vi "Com_Lookup.vi"(8 "Fehler (Eingang, kein Fehler)":errorcluster) -> (0 "Fehler (Ausgang)":errorcluster, 3 "find list":string[](array[string]))   [LabVIEW 2020, in "Linearisierung v2.lvlib" / "Gasteiler.lvlib" / "HovaCAL_Interface.lvlib" / "Helper.lvlib"]
uses:
  Helper.lvlib
  <vilib>/Instr/_visa.llb/VISA Find Search Mode.ctl
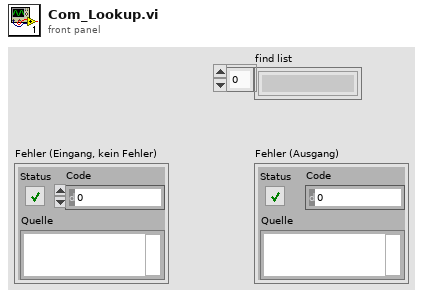
[diagram p1: front panel]
types:
  T1 = typedef "VISA Find Search Mode.ctl" = u32
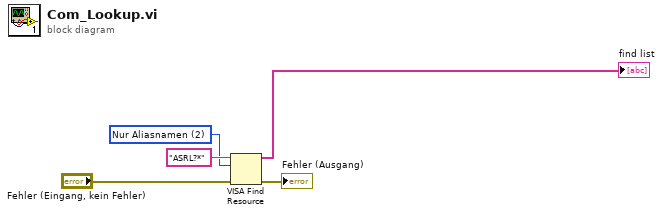
[diagram p0: block diagram]
diagram:
  w3 = T1 2 items=["Nur anerkannte Namen"=0, "Nur Aliasnamen"=2, "Übereinstimmende Aliasnamen einschließen"=3, "Alle Aliasnamen einschließen"=4] ("Search Mode")
  n1 = VISA Find Resource(8:"Fehler (Eingang, kein Fehler)", 10:w3, 11:"ASRL?*" ("Ausdruck (\"?*\")")) -> (0:→"Fehler (Ausgang)":errorcluster, 3:→"find list":string[])  [unwired: 1 out]
